vi "Embed_Hide.vi"(8 "error in (no error)":errorcluster, 11 "EmbeddedSMO in":refnum<class "SMO.UI.Embedded.lvclass">) -> (0 "error out":errorcluster, 3 "EmbeddedSMO out":refnum<class "SMO.UI.Embedded.lvclass">)   [LabVIEW 2016, in "SMO.UI.Embedded.lvclass"]
uses:
  SMO.UI.Embedded.lvclass
  Typedefs/UI State.ctl
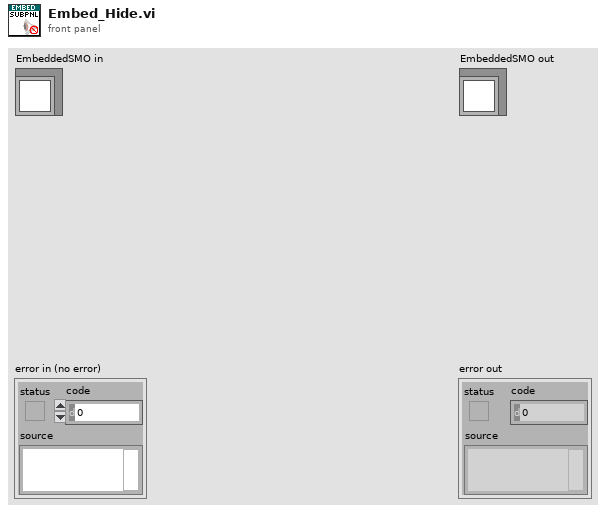
[diagram p1: front panel]
types:
  T1 = typedef "SMO.UI.Embedded.lvclass/UI State.ctl" = enum16{"unknown", "Opened", "Embedded", "Closed"}
  T2 = enum32{"Invalid", "Standard", "Closed", "Hidden", "Minimized", "Maximized"}
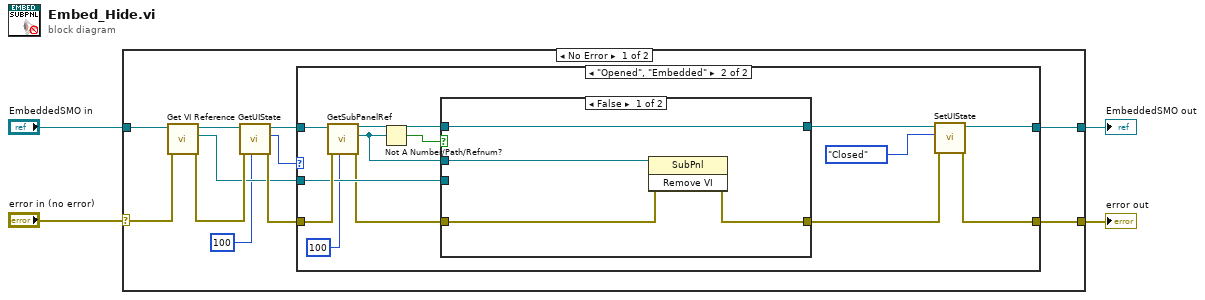
[diagram p0: block diagram]
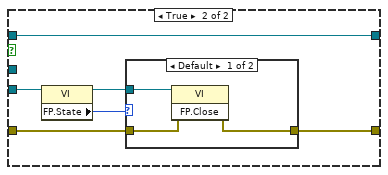
[diagram p3: hidden frame]
diagram:
  n1 = case shown="No Error" "error in (no error)" {
    selector: "error in (no error)" -> [w7 w46]
    tunnel: [w11 w46] -> w3
    tunnel: [w15 w45] -> w1
    tunnel: "EmbeddedSMO in" -> [w10 w45]
    frame No Error {
      n2 = call-dynamic "Get VI Reference.vi"("error in (no error)"=w7, "SMO UI"=w10) -> ("error out"=w8:errorcluster, "VI Reference"=w6:refnum<vi>, "SMO UI out"=w9:refnum<class "SMO.UI.Embedded.lvclass">)  [unwired: 7 in]
      n3 = call "GetUIState.vi"("timeout in ms (-1)"=100, "error in (no error)"=w8, "EmbeddedSMO in"=w9) -> ("error out"=w12:errorcluster, "UI State"=w13:T1, "EmbeddedSMO out"=w14:refnum<class "SMO.UI.Embedded.lvclass">)  [unwired: 6 in]
      n4 = case shown="\"Opened\", \"Embedded\"" w13 {
        tunnel: w14 -> [w17 w30]
        tunnel: [w17 w24] -> w15
        tunnel: w6 -> [_ w26]
        tunnel: w12 -> [w16 w29]
        tunnel: [w16 w20] -> w11
        frame Default {
        }
        frame "Opened", "Embedded" {
          n5 = call "GetSubPanelRef.vi"("timeout in ms (-1)"=100, "error in (no error)"=w29, "EmbeddedSMO in"=w30) -> ("error out"=w21:errorcluster, "SubPanelReference"=w25:refnum<vi>, "EmbeddedSMO out"=w28:refnum<class "SMO.UI.Embedded.lvclass">)  [unwired: 6 in]
          n6 = Not A Number/Path/Refnum?(number/path/refnum=w25) -> (NaN/Path/Refnum?=w27:bool)
          n7 = case shown="False" w27 {
            tunnel: w28 -> [w34 w40]
            tunnel: [w34 w40] -> w23
            tunnel: w26 -> [_ w37]
            tunnel: w25 -> [w33 _]
            tunnel: [w31 w38] -> w22
            tunnel: w21 -> [w32 w39]
            frame False {
              n8 = invoke class="SubPnl" method="Remove VI"(reference=w33, error in=w32) -> (error out=w31:errorcluster)  [unwired: 1 in, 2 out]
            }
            frame True {
              n9 = property class="VI"(reference=w37) -> (reference out=w36:refnum<vi>, "FP.State"=w35:T2)  [unwired: 1 in, 1 out]
              n10 = case shown="Default" w35 {
                tunnel: w39 -> [w43 w44]
                tunnel: [w42 w44] -> w38
                tunnel: w36 -> [w41 _]
                frame Default {
                  n11 = invoke class="VI" method="FP.Close"(reference=w41, error in=w43) -> (error out=w42:errorcluster)  [unwired: 1 in, 2 out]
                }
                frame "Closed" {
                }
              }
            }
          }
          n12 = call "SetUIState.vi"("error in (no error)"=w22, "UI State"=UI_State."Closed", "EmbeddedSMO in"=w23) -> ("error out"=w20:errorcluster, "EmbeddedSMO out"=w24:refnum<class "SMO.UI.Embedded.lvclass">)  [unwired: 7 in]
        }
      }
    }
    frame Error {
    }
  }
  "error out" <- w3
  "EmbeddedSMO out" <- w1
